vi "Write Setpoint (Multiple).vi"(6 "Values":string, 8 "error in (no error)":errorcluster, 9 "Variables":string, 10 "IED Names":string, 11 "SCADA in":refnum<class "SCADA.lvclass">) -> (0 "error out":errorcluster, 3 "SCADA out":refnum<class "SCADA.lvclass">)   [LabVIEW 2015, in "SCADA Core.lvlib" / "SCADA.lvclass"]
uses:
  SCADA.lvclass
  <vilib>/ActorFramework/Actor/Actor.lvclass/Actor.ctl
  <vilib>/ActorFramework/Message Enqueuer/Message Enqueuer.lvclass/Message Enqueuer.ctl
  Controls/Queue Selector.ctl
  SCADA Messages/Multiple Setpoint Setup Msg/Multiple Setpoint Setup Msg.lvclass/Multiple Setpoint Setup Msg.ctl
  SCADA.lvclass/SCADA.ctl
  IED Actor/IED Messages/Write Setpoint Msg/Write Setpoint Msg.lvclass/Write Setpoint Msg.ctl
  SCADA Abstract Messages/IED Setpoint Status Msg/IED Setpoint Status.ctl
  SCADA Response Messages/Return Setpoint Status Msg/Return Setpoint Status Msg.lvclass/Return Setpoint Status Msg.ctl
  <vilib>/ActorFramework/Message Enqueuer/Init from Existing Queue.vi
  <vilib>/ActorFramework/Message Enqueuer/Enqueue.vi
  <vilib>/NI/Tools/Keyed Array/Map String.vi
  <vilib>/NI/Tools/String/Get Case Matching.vi
  <vilib>/ActorFramework/Message Priority Queue/Priority Enqueue.vi
  <vilib>/ActorFramework/Message Enqueuer/Message Enqueuer.lvclass
  SCADA Messages/Multiple Setpoint Setup Msg/Multiple Setpoint Setup Msg.lvclass
  IED Actor/IED Messages/Write Setpoint Msg/Write Setpoint Msg.lvclass
  SCADA Response Messages/Return Setpoint Status Msg/Return Setpoint Status Msg.lvclass
  SCADA Abstract Messages/IED Setpoint Status Msg/IED Setpoint Status Msg.lvclass
  <vilib>/ActorFramework/Actor/Actor.lvclass
  Utilities/Message Strings.llb/Message String Utilities.lvlib
  <vilib>/NI/Tools/Keyed Array/Tools_KeyedArray.lvlib
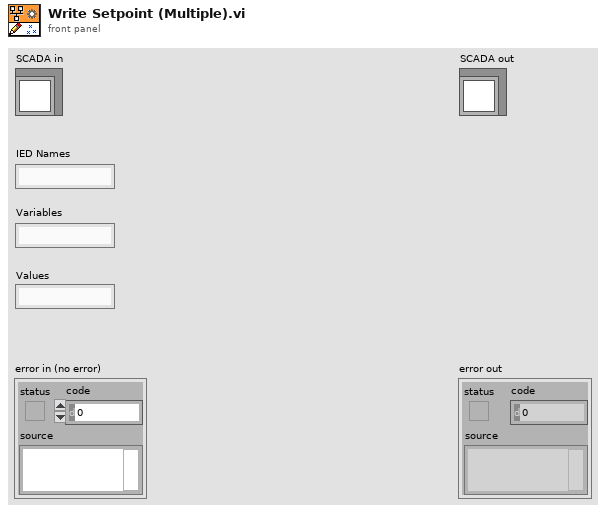
[diagram p1: front panel]
types:
  T1 = typedef "SCADA Core.lvlib/IED Setpoint Status Msg.lvclass/IED Setpoint Status.ctl" = enum16{"Success", "Failure", "Multiple Success", "Multiple Failure"}
  T2 = typedef "SCADA Core.lvlib/SCADA.lvclass/Queue Selector.ctl" = enum16{"IEDs", "PV", "Generators", "Wind", "Storage", "Relays"}
  T3 = typedef "Tools_KeyedArray.lvlib/KeyedArray.ctl" = cluster{"keys":string[], "values":string[]}
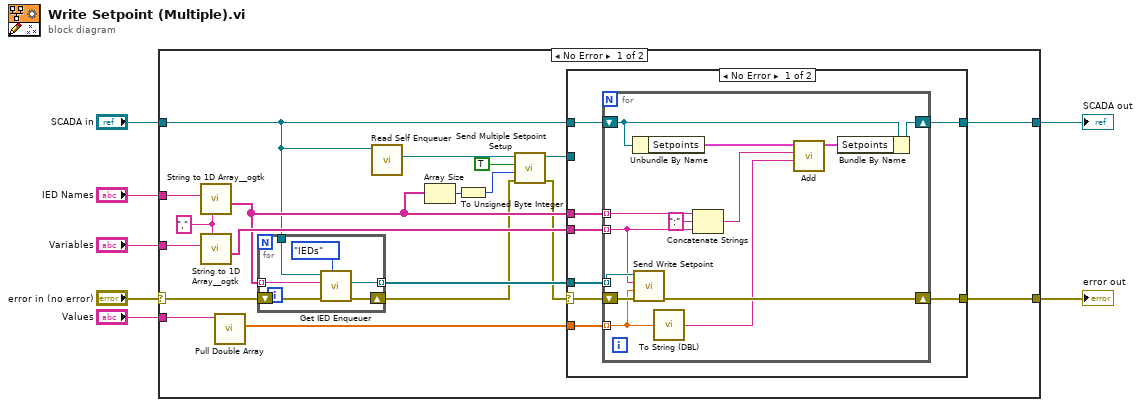
[diagram p0: block diagram]
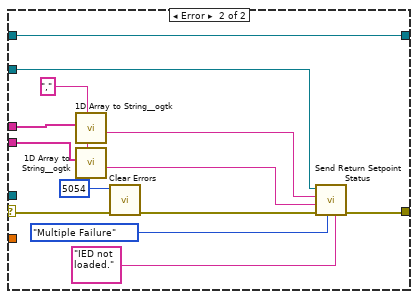
[diagram p2: hidden frame]
diagram:
  n1 = case shown="No Error" "error in (no error)" {
    selector: "error in (no error)" -> [w26 w68]
    tunnel: [w25 w68] -> w6
    tunnel: [w8 w67] -> w4
    tunnel: "SCADA in" -> [w9 w67]
    tunnel: "IED Names" -> [w24 _]
    tunnel: "Variables" -> [w23 _]
    tunnel: "Values" -> [w20 _]
    frame No Error {
      w21 = "," ("delimiter (Tab)")
      n2 = call <userlib>:"String to 1D Array__ogtk.vi"("delimiter (Tab)"=w21, "string"=w24) -> ("Array of Strings"=w14:string[])  [unwired: 9 in]
      n3 = call <userlib>:"String to 1D Array__ogtk.vi"("delimiter (Tab)"=w21, "string"=w23) -> ("Array of Strings"=w22:string[])  [unwired: 9 in]
      n4 = call "Pull Double Array.vi"("String in"=w20) -> ("Array out"=w19:dbl[])  [unwired: 8 in, 2 out]
      n5 = for {
        tunnel: w9 -> [w65]
        tunnel: w14 -> [w64] mode=indexing
        shift-right: [w63] -> w11
        shift-left: w26 -> [w66]
        tunnel: [w61] -> w18 mode=indexing
        n6 = call "Get IED Enqueuer.vi"("Queue (IEDs)"=Queue_Selector."IEDs" ("Queue"), "error in (no error)"=w66, "IED Name"=w64, "SCADA in"=w65) -> ("error out"=w63:errorcluster, "IED Enqueuer"=w61:refnum<class "Message Enqueuer.lvclass">)  [unwired: 5 in, 1 out]
      }
      n7 = call <vilib>:"Read Self Enqueuer.vi"("Actor"=w9) -> ("Self Enqueuer"=w17:refnum<class "Message Enqueuer.lvclass">)  [unwired: 10 in]
      n8 = Array Size(array=w14) -> (size(s)=w13:i32)
      n9 = To Unsigned Byte Integer(number=w13) -> (unsigned 8bit integer=w12:u8)
      n10 = call "Send Multiple Setpoint Setup.vi"("error in (no error)"=w11, "Number of Setpoints"=w12, "Multiple Setpoints?"=TRUE, "Message Enqueuer"=w17) -> ("error out"=w10:errorcluster, "Message Enqueuer out"=w16:refnum<class "Message Enqueuer.lvclass">)  [unwired: 6 in]
      n11 = case shown="No Error" w10 {
        selector: w10 -> [w30 w56]
        tunnel: [w34 w49] -> w25
        tunnel: w14 -> [w27 w54]
        tunnel: w22 -> [w33 w52]
        tunnel: w19 -> [w32 _]
        tunnel: w16 -> [_ w55]
        tunnel: w18 -> [w31 _]
        tunnel: w9 -> [w29 w48]
        tunnel: [w28 w48] -> w8
        frame No Error {
          n12 = for {
            tunnel: w33 -> [w38] mode=indexing
            tunnel: w32 -> [w36] mode=indexing
            tunnel: w31 -> [w47] mode=indexing
            shift-right: [w45] -> w34
            shift-left: w30 -> [w46]
            shift-right: [w43] -> w28
            shift-left: w29 -> [w44]
            tunnel: w27 -> [w39] mode=indexing
            n13 = Unbundle By Name(w44) -> ("Setpoints"=w42:T3)
            n14 = call "Send Write Setpoint.vi"("error in (no error)"=w46, "Value"=w36, "Variable"=w38, "Message Enqueuer"=w47) -> ("error out"=w45:errorcluster)  [unwired: 6 in, 1 out]
            n15 = call "To String (DBL).vi"("Double in"=w36) -> ("String out"=w35:string)
            n16 = Concatenate Strings(w39, ":" ("string"), w38) -> (w37:string)
            n17 = call <vilib>:"Add.vi"("value"=w35, "key"=w37, "array in"=w42) -> ("array out"=w41:T3)  [unwired: 2 in, 2 out]
            n18 = Bundle By Name(cluster=w44, "Setpoints"=w41) -> (w43:refnum<class "SCADA.lvclass">)
          }
        }
        frame Error {
          w51 = "," ("delimiter (Tab)")
          n19 = call <userlib>:"1D Array to String__ogtk.vi"("delimiter (Tab)"=w51, "Array of Strings"=w54) -> ("delimited string"=w53:string)  [unwired: 9 in]
          n20 = call <userlib>:"1D Array to String__ogtk.vi"("delimiter (Tab)"=w51, "Array of Strings"=w52) -> ("delimited string"=w50:string)  [unwired: 9 in]
          n21 = call <vilib>:"Clear Errors.vi"("error in (no error)"=w56, "specific error code to clear (0: all)"=5054) -> ("error out"=w60:errorcluster)  [unwired: 4 in, 1 out]
          n22 = call "Send Return Setpoint Status.vi"("error"="IED not loaded." ("Error String"), "Status"=IED_Setpoint_Status."Multiple Failure", "error in (no error)"=w60, "Setpoint Name"=w50, "IED Name"=w53, "Message Enqueuer"=w55) -> ("error out"=w49:errorcluster)  [unwired: 4 in, 1 out]
        }
      }
    }
    frame Error {
    }
  }
  "error out" <- w6
  "SCADA out" <- w4
